vi "PID_position.vi"() -> ()   [LabVIEW 2014]
uses:
  <vilib>/FPGAPlugInAG/cRIO-9068/niLvFpga_Open_cRIO-9068.vi
  <vilib>/rvi/interface/common/dynamic/niFpgaDynamicAddResources.vi
  <vilib>/Utility/error.llb/Error Cluster From Error Code.vi
  <vilib>/rvi/errors/niLvFpgaAdjustHostInterfaceError.vi
  <vilib>/addons/control/pid/pid.llb/PID (DBL).vi
  <vilib>/FPGAPlugInAG/Dynamic/niLvFpga_Close_Dynamic.vi
  <vilib>/rvi/interface/nirviOpenFPGA/nirviOpenFPGA.xnode
  FPGA Bitfiles/Motortest_FPGATarget_test6auto_Jx62XASY7Q8.lvbitx
  <vilib>/rvi/interface/nirviReadWriteControl/nirviReadWriteControl.xnode
  <vilib>/rvi/interface/nirviCloseFPGA/nirviCloseFPGA.xnode
  NiFpgaLv.dll
  <vilib>/rvi/interface/Simulation/niFpgaSimulationCallBeginRW.vi
  <vilib>/addons/control/pid/NI_PID_pid.lvlib
panel:
  out "Duty Cycle":cluster{dbl[], dbl[]}(graph)
  out "Velocity [Revolution/second]":cluster{dbl[], sgl[]}(graph)
  out "Position [Revolution]":cluster{dbl[], sgl[]}(graph)
  out "Velocity Setpoint [Revolution/second]":cluster{dbl[], dbl[]}(graph)
  out "Velocity Setpoint":dbl[](graph)
  out "Position":sgl[](graph)
  in  "PID Position":T1={"proportional gain (Kc)"=2.0, "integral time (Ti, min)"=0.0, "derivative time (Td, min)"=0.0} {"derivative time (Td, min)" format="%.3f"; "integral time (Ti, min)" format="%.3f"; "proportional gain (Kc)" format="%.3f"}
  in  "Desired Position\n[Rounds]":dbl=500.0
  in  "stop":bool
  out "Position [Round]":sgl
  out "Velocity [RPS]":sgl
  in  "PID gains":T1={"proportional gain (Kc)"=0.15, "integral time (Ti, min)"=0.0002, "derivative time (Td, min)"=0.0} {"derivative time (Td, min)" format="%.4f"; "integral time (Ti, min)" format="%.4f"; "proportional gain (Kc)" format="%.4f"}
  in  "output range":cluster{"output high":dbl, "output low":dbl}={"output high"=100.0, "output low"=-100.0} {"output low" format="%.2f"; "output high" format="%.2f"}
  out "Duty Cycle":dbl format="%.2f"
  out "Velocity":sgl[](graph)
  out "Error":dbl(slide) scale=0.0..50.0
  out "Duty Cycle 2":dbl(slide) scale=0.0..1.0
  out "Duty Cycle":dbl[](graph)
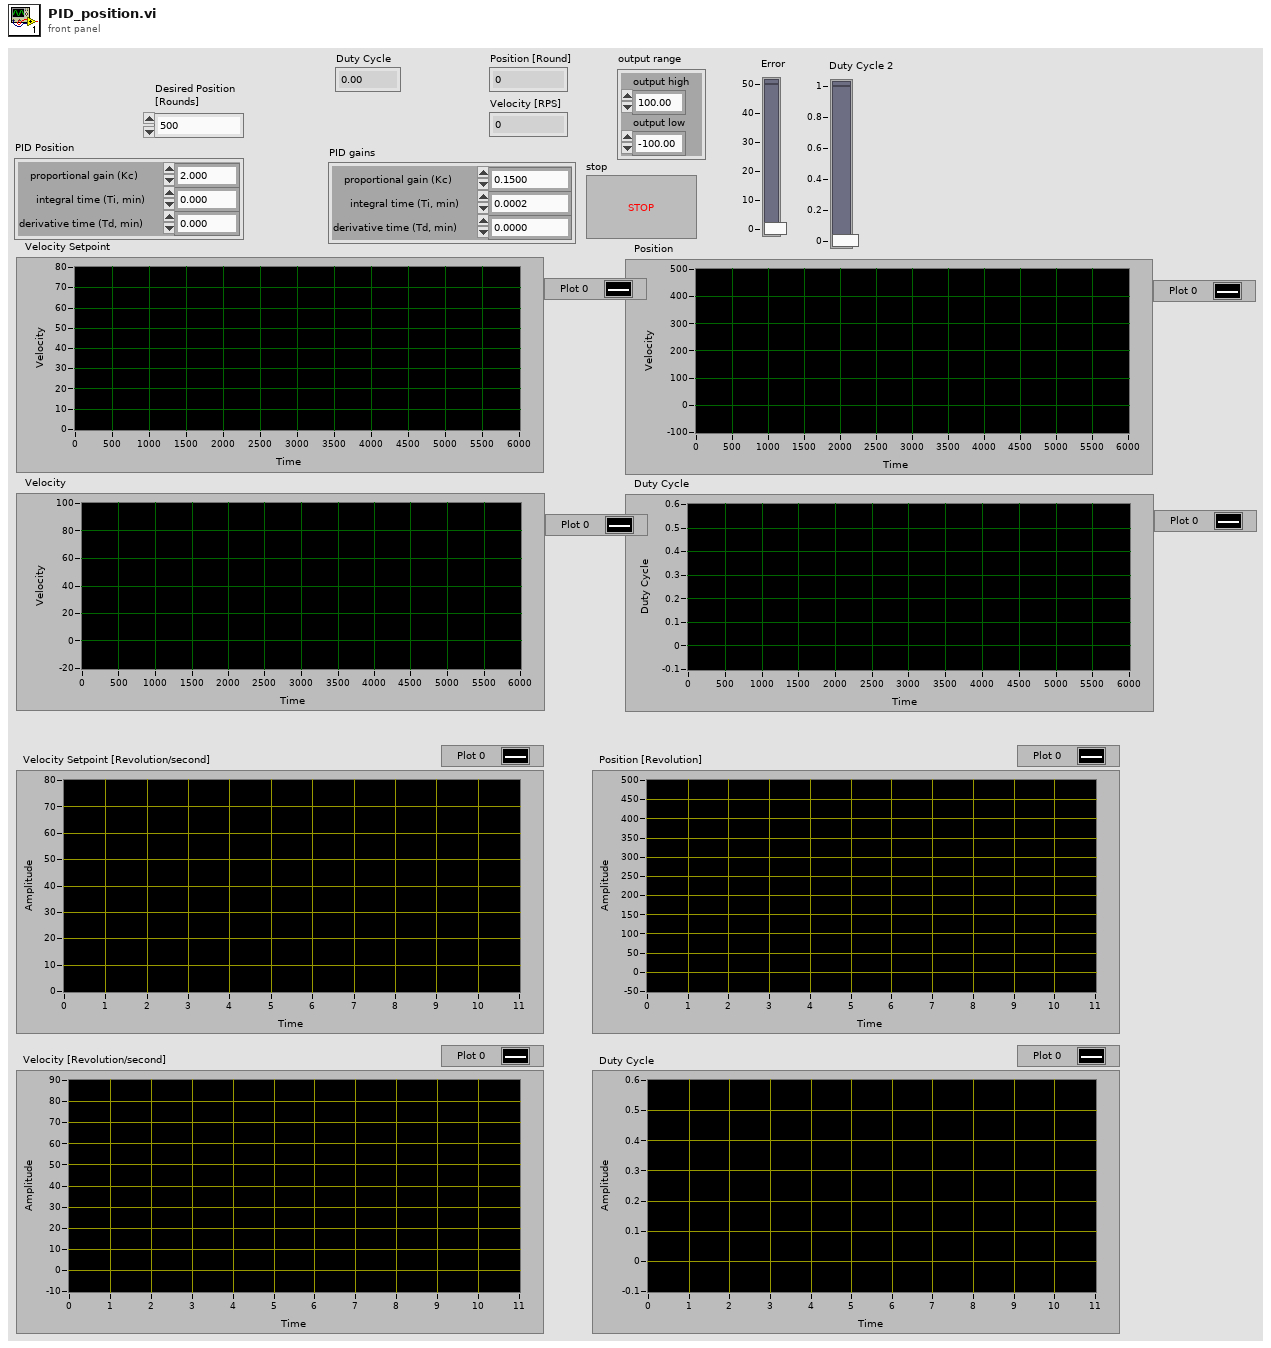
[diagram p1: front panel]
types:
  T1 = cluster{"proportional gain (Kc)":dbl, "integral time (Ti, min)":dbl, "derivative time (Td, min)":dbl}
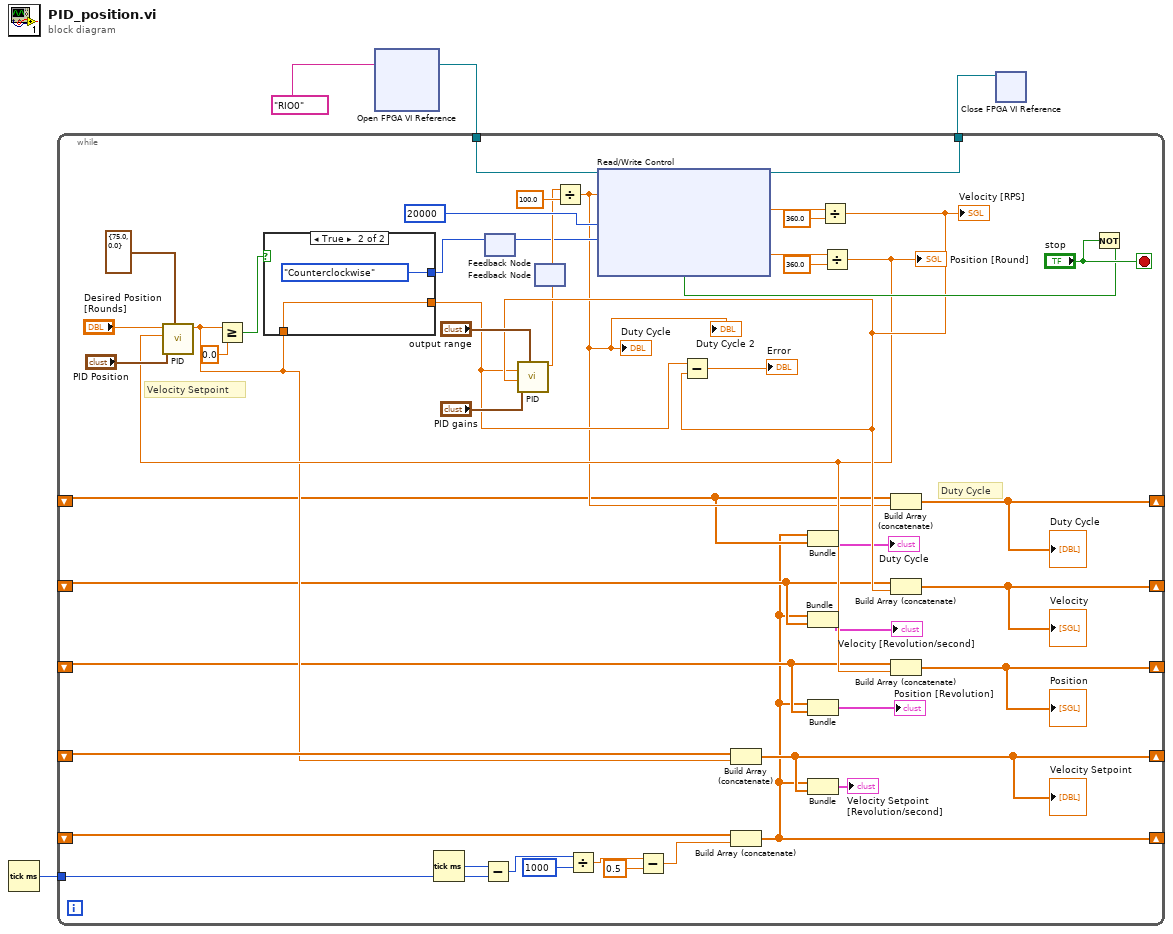
[diagram p0: block diagram]
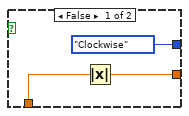
[diagram p2: hidden frame]
diagram:
  n1 = Tick Count (ms)() -> (millisecond timer value=w1:u32)
  n2 = xnode "Open FPGA VI Reference"("resource name"=tag "RIO0") -> ("FPGA VI Reference Out"=w2:refnum<k20>)  [unwired: 1 in, 1 out]
  n3 = while {
    tunnel: w2 -> [w52]
    tunnel: [w51] -> w4
    shift-right: [w37] -> _
    shift-left: _ -> [w10]
    shift-right: [w38] -> _
    shift-left: _ -> [w6]
    shift-right: [w30] -> _
    shift-left: _ -> [w9]
    shift-right: [w12] -> _
    shift-left: _ -> [w24]
    shift-right: [w5] -> _
    shift-left: _ -> [w21]
    tunnel: w1 -> [w19]
    stop <- "stop" stop-if-true
    # "Velocity Setpoint"
    # "Duty Cycle"
    n4 = Tick Count (ms)() -> (millisecond timer value=w18:u32)
    n5 = Subtract(x=w18, y=w19) -> (x-y=w17:u32)
    n6 = feedback #1() -> (w26:enum8{"Clockwise", "Counterclockwise"})  [unwired: 1 in]
    n7 = feedback #2() -> (w35:dbl)  [unwired: 1 in]
    n8 = Divide(x=w35, y=100.0) -> (x/y=w22:dbl)
    "Duty Cycle" <- w22
    "Duty Cycle 2" <- w22
    n9 = Divide(x=w17, y=u32 1000) -> (x/y=w15:dbl)
    n10 = Subtract(x=w15, y=0.5) -> (x-y=w16:dbl)
    n11 = Build Array (concatenate)(w21, w16) -> (w5:dbl[])
    n12 = Bundle(w5, w10) -> (→"Duty Cycle":cluster{dbl[], dbl[]})  [unwired: 1 in]
    n13 = Bundle(w5, w6) -> (→"Velocity [Revolution/second]":cluster{dbl[], sgl[]})  [unwired: 1 in]
    n14 = Bundle(w5, w9) -> (→"Position [Revolution]":cluster{dbl[], sgl[]})  [unwired: 1 in]
    n15 = Build Array (concatenate)(w10, w22) -> (w37:dbl[])
    "Duty Cycle" <- w37
    n16 = Not(x="stop") -> (.not. x?=w49:bool)
    n17 = xnode "Read/Write Control"("FPGA VI Reference In"=w52, "duty cycle (periods)"=w22, "Velocity Interval (uSec)"=u32 20000, "Mod1/Drive Direction"=w26, "Mod1/Motor"=w49) -> ("FPGA VI Reference Out"=w51:refnum<k20>, "Velocity (Degrees/Second)"=w42:sgl, "Position (Degrees)"=w45:sgl)  [unwired: 1 in, 1 out]
    n18 = Divide(x=w42, y=sgl 360.0) -> (x/y=w40:sgl)
    "Velocity [RPS]" <- w40
    n19 = Divide(x=w45, y=sgl 360.0) -> (x/y=w31:sgl)
    "Position [Round]" <- w31
    n20 = call-poly <vilib>:"PID.vi"("output range"=cluster{"output high":dbl, "output low":dbl} {"output high"=75.0, "output low"=0.0}, "PID gains"="PID Position", "process variable"=w31, "setpoint"="Desired Position\n[Rounds]") -> ("output"=w23:dbl)  [unwired: 6 in, 1 out]
    n21 = Greater Or Equal?(x=w23, y=0.0) -> (x >= y?=w28:bool)
    n22 = case shown="True" w28 {
      tunnel: [enum8{"Clockwise", "Counterclockwise"}."Clockwise" ("Mod1/Drive Direction") enum8{"Clockwise", "Counterclockwise"}."Counterclockwise" ("Mod1/Drive Direction")] -> w27
      tunnel: w23 -> [w54 w56]
      tunnel: [w53 w56] -> w25
      frame False {
        n23 = Absolute Value(x=w54) -> (abs(x)=w53:dbl)
      }
      frame True {
      }
    }
    n24 = feedback-in #1(w27) -> ()
    n25 = call-poly <vilib>:"PID.vi"("output range"="output range", "PID gains"="PID gains", "process variable"=w40, "setpoint"=w25) -> ("output"=w36:dbl)  [unwired: 6 in, 1 out]
    n26 = feedback-in #2(w36) -> ()
    n27 = Subtract(x=w25, y=w40) -> (x-y=→"Error":dbl)
    n28 = Build Array (concatenate)(w24, w23) -> (w12:dbl[])
    "Velocity Setpoint" <- w12
    n29 = Bundle(w5, w12) -> (→"Velocity Setpoint [Revolution/second]":cluster{dbl[], dbl[]})  [unwired: 1 in]
    n30 = Build Array (concatenate)(w6, w40) -> (w38:sgl[])
    "Velocity" <- w38
    n31 = Build Array (concatenate)(w9, w31) -> (w30:sgl[])
    "Position" <- w30
  }
  n32 = xnode "Close FPGA VI Reference"("FPGA VI Reference In"=w4) -> ()  [unwired: 1 in, 1 out]
